vi "autoCoag.vi"(6 "state":T3, 7 "current time":timestamp, 8 "error in (no error)":errorcluster, 10 "data input":T2) -> (0 "error out":errorcluster, 1 "coag model":T1, 2 "total HRT":dbl)   [LabVIEW 2015]
uses:
  <vilib>/Utility/config.llb/NI_LVConfig.lvlib
  Sensor buffer command.ctl
  <vilib>/Utility/config.llb/Write Key (String).vi
  data cluster.ctl
  <vilib>/Utility/config.llb/Read Key (String).vi
  calcDoseorGetGraph.ctl
  ini.ctl
  coagbuffer.ctl
  state.ctl
  model type.ctl
  coag model data.ctl
panel:
  out "length":i32
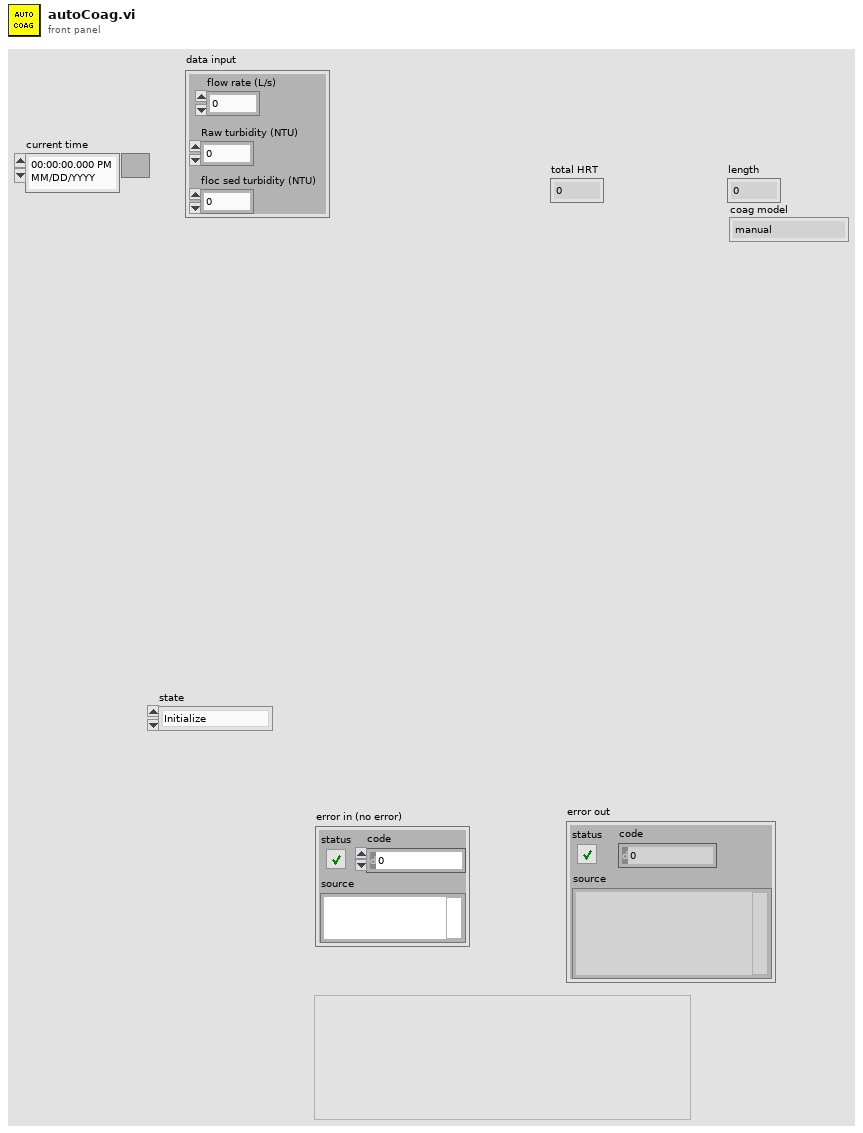
[diagram p1: front panel]
types:
  T1 = typedef "model type.ctl" = enum16{"manual", "ramp", "simple corrector", "linear regression"}
  T2 = typedef "coag model data.ctl" = cluster{"flow rate (L/s)":dbl, "Raw turbidity (NTU)":dbl, "floc sed turbidity (NTU)":dbl}
  T3 = typedef "state.ctl" = enum16{"Initialize", "Process data", "Close"}
  T4 = typedef "ini.ctl" = enum16{"write", "read"}
  T5 = typedef "coagbuffer.ctl" = enum16{"set buffer size", "write", "refill buffer", "read recent", "read all", "clear", "overwrite"}
  T6 = typedef "Sensor buffer command.ctl" = enum16{"set buffer size", "write", "refill buffer", "read recent", "read all", "clear"}
  T7 = typedef "data cluster.ctl" = cluster{"floc sed turbidity (NTU)":dbl, "Raw turbidity (NTU)":dbl, "flow rate (L/s)":dbl, "time":timestamp}
  T8 = typedef "calcDoseorGetGraph.ctl" = enum16{"calculate dose", "read graph"}
  T9 = typedef "setpoints.ctl" = cluster{"graph data interval (s)":sgl, "sludge flow [L/s]":dbl, "plant flow [L/s]":dbl, "Plant Flow PID ":cluster{"proportional gain (Kc)":dbl, "integral time (Ti, min)":dbl, "derivative time (Td, min)":dbl}, "Sludge PID ":cluster{"proportional gain (Kc)":dbl, "integral time (Ti, min)":dbl, "derivative time (Td, min)":dbl}, "backwash":T10, "Coagulant":T11}
  T10 = typedef "backwash.ctl" = cluster{"Filtered quality target [NTU]":dbl, "min filtration time [s]":dbl, "Ripen time [s]":dbl}
  T11 = typedef "coag.ctl" = cluster{"flocculator volume (L)":dbl, "clarifier volume (L)":dbl, "dose updates per HRT":u16, "target clarified turbidity (NTU)":dbl, "Coagulant mode":T1, "Coag dose [mg/L]":dbl, "pump mL/rev":dbl, "clarifier flow [L/s]":dbl, "min Coag dose [mg/L]":dbl, "max Coag dose [mg/L]":dbl, "Steps":u16, "HRT response delay":u32, "Ku*":dbl}
  T12 = typedef "NI_LVConfig.lvlib/Config Data RefNum.ctl" = refnum<k1>
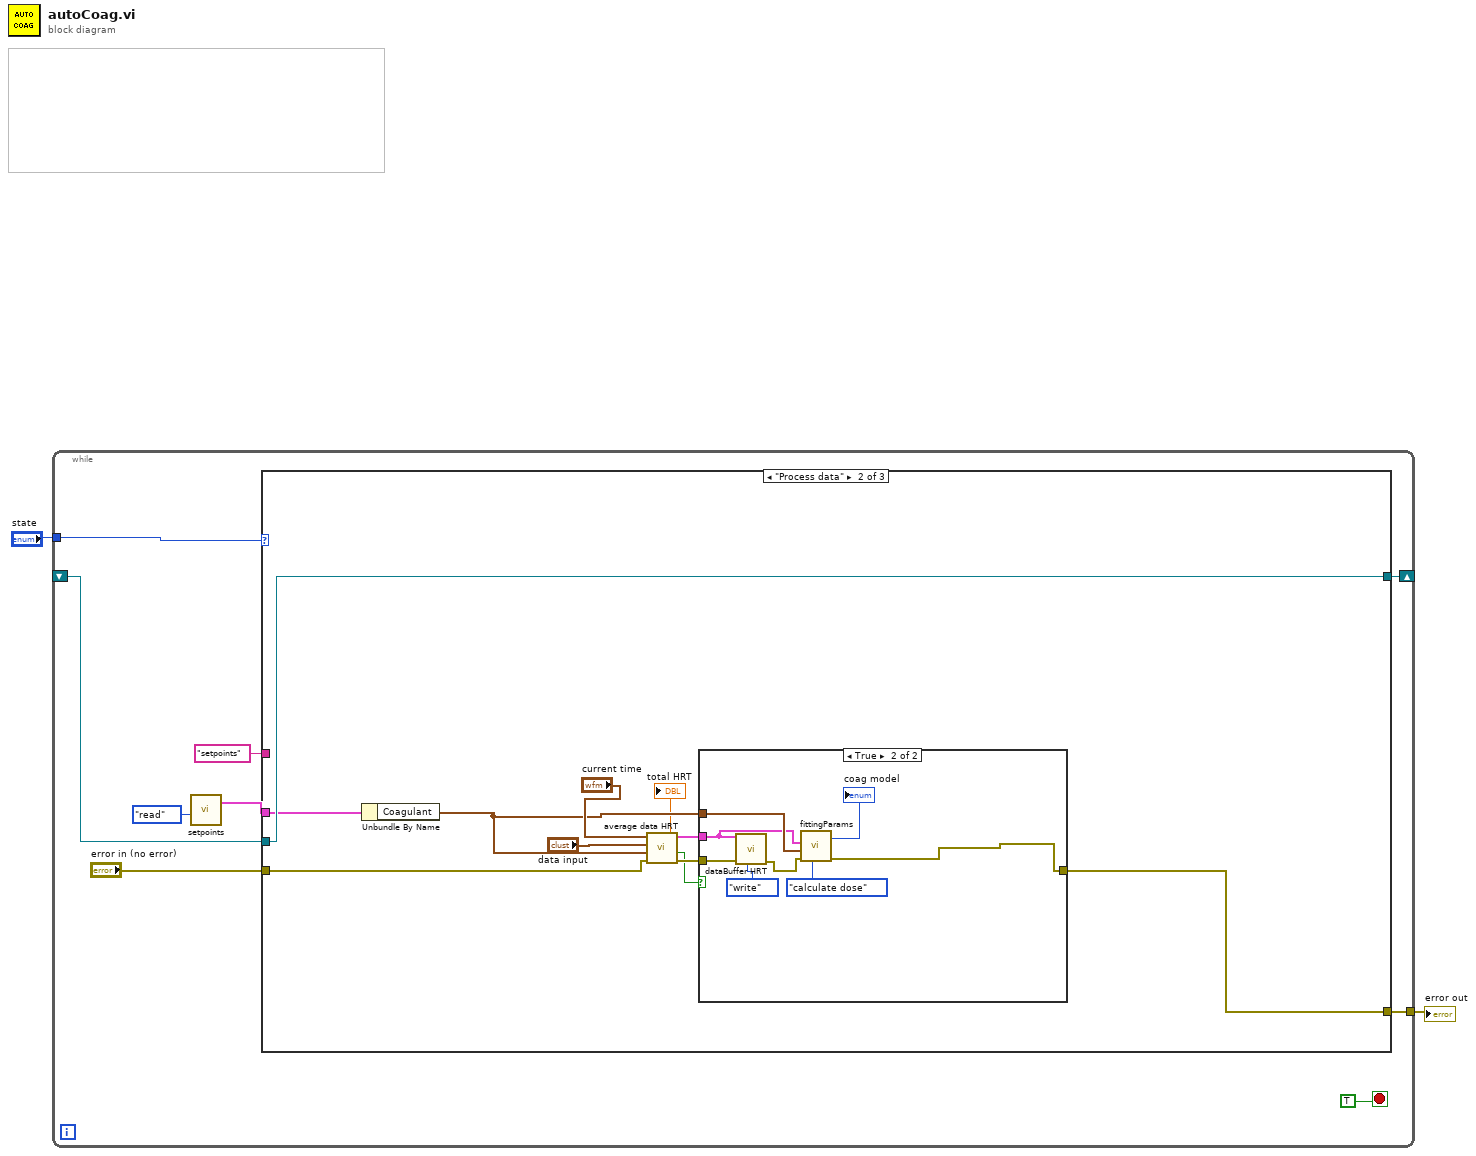
[diagram p0: block diagram]
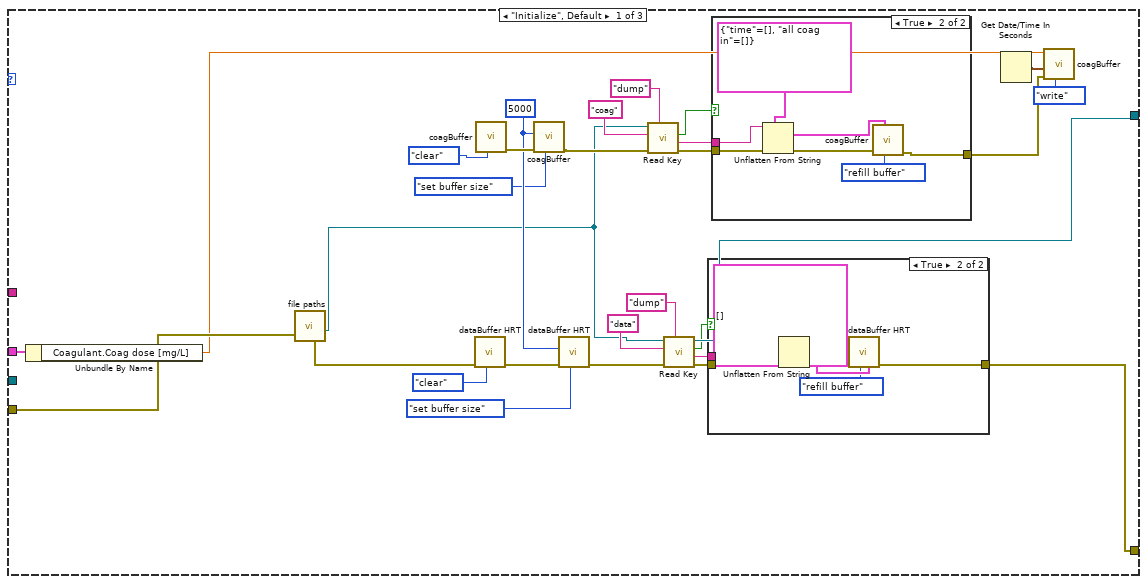
[diagram p2: hidden frame]
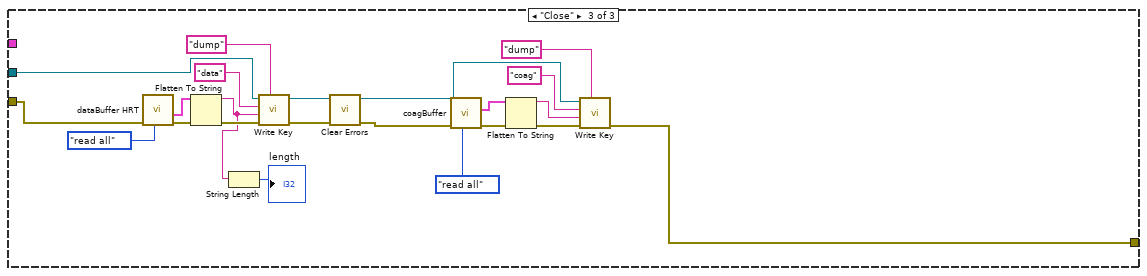
[diagram p6: hidden frame]
diagram:
  n1 = while {
    tunnel: "state" -> [w10]
    shift-right: [w9] -> _
    shift-left: _ -> [w8]
    tunnel: [w6] -> w1
    stop <- TRUE stop-if-true
    n2 = call "setpoints.vi"("ini"=ini."read") -> ("Setpoints out"=w4:T9)  [unwired: 9 in, 1 out]
    n3 = case shown="\"Process data\"" w10 {
      tunnel: [w32 w67 _] -> w9
      tunnel: w8 -> [_ w67 w96]
      tunnel: w4 -> [w15 w57 _]
      tunnel: "setpoints" ("section") -> [_ _ _]
      tunnel: [w17 w62 w78] -> w6
      tunnel: "error in (no error)" -> [w19 w64 w94]
      frame "Initialize", Default {
        w28 = u16 5000 ("max array size")
        n4 = Unbundle By Name(w15) -> ("Coagulant.Coag dose [mg/L]"=w14:dbl)
        n5 = call "file paths.vi"("error in (no error)"=w19) -> ("ini"=w20:T12, "error out"=w18:errorcluster)  [unwired: 7 in, 2 out]
        n6 = call "dataBuffer HRT.vi"("command"=Sensor_buffer_command."clear", "error in (no error)"=w18) -> ("error out"=w38:errorcluster)  [unwired: 6 in, 3 out]
        n7 = call "coagBuffer.vi"("command"=Sensor_buffer_command."clear") -> ("error out"=w29:errorcluster)  [unwired: 8 in, 2 out]
        n8 = call "coagBuffer.vi"("command"=Sensor_buffer_command."set buffer size", "error in (no error)"=w29, "max array size"=w28) -> ("error out"=w21:errorcluster)  [unwired: 6 in, 2 out]
        n9 = call "dataBuffer HRT.vi"("command"=Sensor_buffer_command."set buffer size", "error in (no error)"=w38, "max array size"=w28) -> ("error out"=w35:errorcluster)  [unwired: 5 in, 3 out]
        n10 = call-poly <vilib>:"Read Key.vi"("section"="dump", "error in (no error)"=w21, "key"="coag", "refnum"=w20) -> ("error out"=w24:errorcluster, "value"=w25:string, "found?"=w26:bool)  [unwired: 4 in, 1 out]
        n11 = call-poly <vilib>:"Read Key.vi"("section"="dump", "error in (no error)"=w35, "key"="data", "refnum"=w20) -> ("error out"=w34:errorcluster, "value"=w33:string, "found?"=w31:bool, "refnum out"=w32:T12)  [unwired: 4 in]
        n12 = case shown="True" w31 {
          tunnel: w34 -> [w49 w56]
          tunnel: w33 -> [_ w55]
          tunnel: [w49 w50] -> w17
          frame False {
          }
          frame True {
            n13 = Unflatten From String(type=T7[] [] ("all data out"), binary string=w55, error in (no error)=w56) -> (value=w53:T7[], error out=w51:errorcluster)  [unwired: 2 in, 1 out]
            n14 = call "dataBuffer HRT.vi"("all data in"=w53, "command"=Sensor_buffer_command."refill buffer", "error in (no error)"=w51) -> ("error out"=w50:errorcluster)  [unwired: 5 in, 3 out]
          }
        }
        n15 = case shown="True" w26 {
          tunnel: w24 -> [w41 w48]
          tunnel: w25 -> [_ w47]
          tunnel: [w41 w42] -> w12
          frame False {
          }
          frame True {
            n16 = Unflatten From String(type=cluster{"time":timestamp[], "all coag in":dbl[]} {"time"=[], "all coag in"=[]} ("all data in"), binary string=w47, error in (no error)=w48) -> (value=w44:cluster{"time":timestamp[], "all coag in":dbl[]}, error out=w46:errorcluster)  [unwired: 2 in, 1 out]
            n17 = call "coagBuffer.vi"("command"=Sensor_buffer_command."refill buffer", "all data in"=w44, "error in (no error)"=w46) -> ("error out"=w42:errorcluster)  [unwired: 6 in, 2 out]
          }
        }
        n18 = Get Date/Time In Seconds() -> (seconds since 1Jan1904=w13:timestamp)
        n19 = call "coagBuffer.vi"("command"=coagbuffer."write", "error in (no error)"=w12, "Time Stamp"=w13, "Coag dose"=w14) -> ()  [unwired: 5 in, 3 out]
      }
      frame "Process data" {
        n20 = Unbundle By Name(w57) -> ("Coagulant"=w59:T11)
        n21 = call "average data HRT.vi"("error in (no error)"=w64, "Coagulant"=w59, "data input"="data input", "seconds since 1Jan1904"="current time") -> ("error out"=w63:errorcluster, "new interval"=w61:bool, "total HRT"=→"total HRT":dbl, "averaged data"=w65:T7)  [unwired: 4 in]
        n22 = case shown="True" w61 {
          tunnel: w65 -> [_ w69]
          tunnel: w63 -> [w68 w75]
          tunnel: [w68 w71] -> w62
          tunnel: w59 -> [_ w73]
          frame False {
          }
          frame True {
            n23 = call "dataBuffer HRT.vi"("command"=Sensor_buffer_command."write", "error in (no error)"=w75, "averaged data"=w69) -> ("error out"=w74:errorcluster)  [unwired: 5 in, 3 out]
            n24 = call "fittingParams.vi"("read/write"=calcDoseorGetGraph."calculate dose", "error in (no error)"=w74, "Coagulant"=w73, "averaged data"=w69) -> ("error out"=w71:errorcluster, "coag model"=→"coag model":T1)  [unwired: 5 in, 1 out]
          }
        }
      }
      frame "Close" {
        n25 = call "dataBuffer HRT.vi"("command"=Sensor_buffer_command."read all", "error in (no error)"=w94) -> ("error out"=w93:errorcluster, "all data out"=w95:T7[])  [unwired: 6 in, 2 out]
        n26 = Flatten To String(anything=w95, error in (no error)=w93) -> (data string=w80:string, error out=w92:errorcluster)  [unwired: 2 in, 1 out]
        n27 = String Length(string=w80) -> (length=→"length":i32)
        n28 = call-poly <vilib>:"Write Key.vi"("section"="dump", "error in (no error)"=w92, "value"=w80, "key"="data", "refnum"=w96) -> ("error out"=w82:errorcluster, "refnum out"=w83:T12)  [unwired: 4 in, 1 out]
        n29 = call <vilib>:"Clear Errors.vi"("error in (no error)"=w82) -> ("error out"=w81:errorcluster)  [unwired: 5 in, 1 out]
        n30 = call "coagBuffer.vi"("command"=Sensor_buffer_command."read all", "error in (no error)"=w81) -> ("error out"=w88:errorcluster, "all data out"=w77:cluster{"time":timestamp[], "all coag in":dbl[]})  [unwired: 7 in, 1 out]
        n31 = Flatten To String(anything=w77, error in (no error)=w88) -> (data string=w85:string, error out=w84:errorcluster)  [unwired: 2 in, 1 out]
        n32 = call-poly <vilib>:"Write Key.vi"("section"="dump", "error in (no error)"=w84, "value"=w85, "key"="coag", "refnum"=w83) -> ("error out"=w78:errorcluster)  [unwired: 4 in, 2 out]
      }
    }
  }
  "error out" <- w1
